vi "Configure Output.vi"(6 "Curent Level (0.0 V)":dbl caption="Voltage Level (0 V)" format="%.2f", 8 "error in (no error)":errorcluster, 9 "Voltage Level (0.0 V)":dbl caption="Voltage Level (0 V)" format="%.2f", 10 "Channel (0: 30V Channel)":T1 caption="Channel (0: +6V)" items=["30V/3A Channel", "30V/3A Channel", "5V/3A Channel"], 11 "VISA resource name":refnum<visa-resource-name>) -> (0 "error out":errorcluster, 3 "VISA resource name out":refnum<visa-resource-name>)   [LabVIEW 2020, in "Library Instrument & Equipement.lvlib" / "Library Power_Supply.lvlib" / "RIGOL DP800 Series.lvlib"]
doc: "Configures output voltage level, channel, and enables or disables the output of the power supply."
uses:
  RIGOL DP800 Series.lvlib
  Channels.ctl
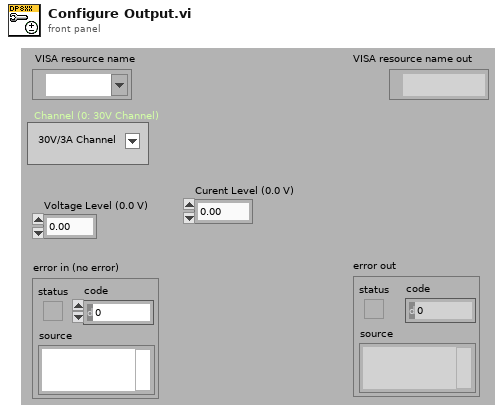
[diagram p1: front panel]
types:
  T1 = typedef "Library Instrument & Equipement.lvlib/Library Power_Supply.lvlib/RIGOL DP800 Series.lvlib/Channels.ctl" = i32
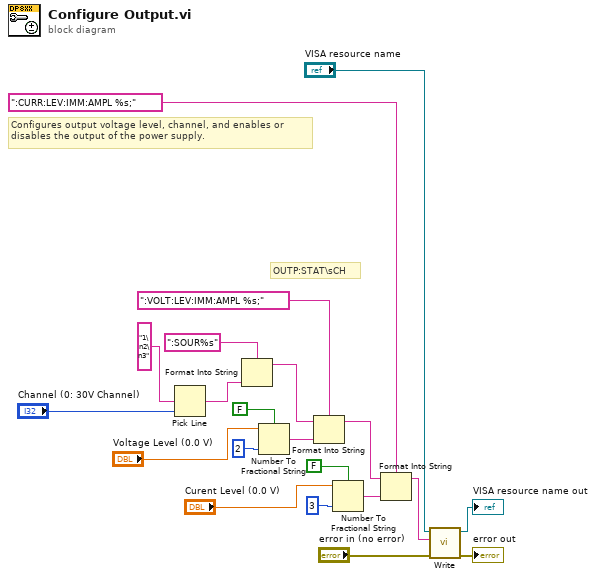
[diagram p0: block diagram]
diagram:
  # "OUTP:STAT\\sCH"
  # "Configures output voltage level, channel, and enables or \ndisables the output of the power supply."
  n1 = Pick Line(multi-line string="1\n2\n3", line index="Channel (0: 30V Channel)") -> (output string=w17:string)  [unwired: 1 out]
  n2 = Format Into String(format string=":SOUR%s", w17) -> (resulting string=w10:string)  [unwired: 2 in, 1 out]
  n3 = Number To Fractional String(use system decimal point (T)=FALSE ("utiliser le séparateur décimal du système (V)"), number="Voltage Level (0.0 V)", precision (6)=i16 2 ("précision (6)")) -> (F-format string=w7:string)  [unwired: 1 in]
  n4 = Format Into String(format string=":VOLT:LEV:IMM:AMPL %s;", initial string=w10, w7) -> (resulting string=w11:string)  [unwired: 1 in, 1 out]
  n5 = Number To Fractional String(use system decimal point (T)=FALSE ("utiliser le séparateur décimal du système (V)"), number="Curent Level (0.0 V)", precision (6)=i16 3 ("précision (6)")) -> (F-format string=w2:string)  [unwired: 1 in]
  n6 = Format Into String(format string=":CURR:LEV:IMM:AMPL %s;", initial string=w11, w2) -> (resulting string=w1:string)  [unwired: 1 in, 1 out]
  n7 = call "Write.vi"("error in (no error)"="error in (no error)", "Write Buffer (\"\")"=w1, "VISA resource name"="VISA resource name") -> ("error out"=→"error out":errorcluster, "VISA resource name out"=→"VISA resource name out":refnum<visa-resource-name>)  [unwired: 7 in]
